vi "Release.vi"(8 "error in":errorcluster, 11 "Lv Proj Document Type:TAF Proj":refnum<class "TAF Proj.lvclass">) -> (0 "error out":errorcluster)   [LabVIEW 2021, in "TAF Proj Document Type.lvlib" / "TAF Proj.lvclass"]
uses:
  <vilib>/Wovalab/AntiDoc/Document Type/Add-ons/LabVIEW TAF Project/TAF Proj/TAF Proj.lvclass
  <vilib>/Wovalab/AntiDoc/Document Type/Add-ons/LabVIEW TAF Project/TAF Proj/TAF Proj.lvclass/TAF Proj.ctl
  <vilib>/Wovalab/AntiDoc/Document Type/Document/Document Type.lvclass
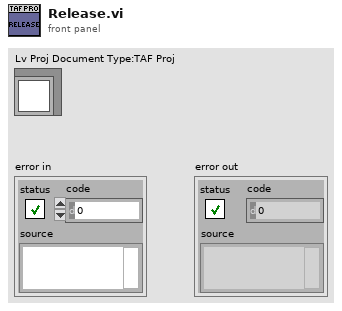
[diagram p1: front panel]
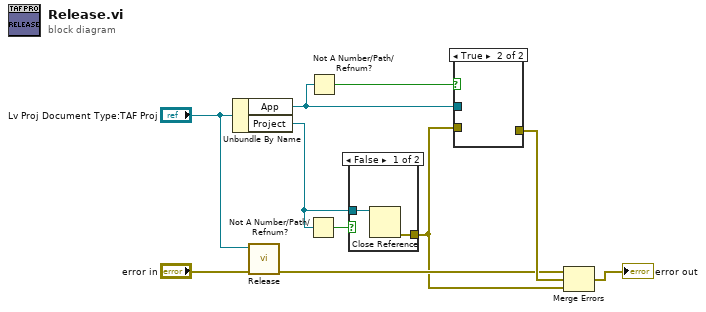
[diagram p0: block diagram]
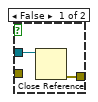
[diagram p3: hidden frame]
diagram:
  n1 = Unbundle By Name("Lv Proj Document Type:TAF Proj") -> ("App"=w5:refnum<vi>, "Project"=w2:refnum<vi>)
  n2 = call-parent "Release.vi"("error in (no error)"="error in", "Document in"="Lv Proj Document Type:TAF Proj") -> ("error out"=w7:errorcluster)  [unwired: 9 in]
  n3 = Not A Number/Path/Refnum?(number/path/refnum=w2) -> (NaN/Path/Refnum?=w3:bool)
  n4 = Not A Number/Path/Refnum?(number/path/refnum=w5) -> (NaN/Path/Refnum?=w4:bool)
  n5 = case shown="False" w3 {
    tunnel: [w12 _] -> w1
    tunnel: w2 -> [w11 _]
    frame False {
      n6 = Close Reference(reference=w11) -> (error out=w12:errorcluster)  [unwired: 1 in]
    }
    frame True {
    }
  }
  n7 = case shown="True" w4 {
    tunnel: [w14 _] -> w9
    tunnel: w5 -> [w13 _]
    tunnel: w1 -> [_ _]
    frame False {
      n8 = Close Reference(reference=w13) -> (error out=w14:errorcluster)  [unwired: 1 in]
    }
    frame True {
    }
  }
  n9 = Merge Errors(w7, w9, w1) -> (→"error out":errorcluster)
